vi "iFlex Open Lines.vi"(8 "error in (no error)":errorcluster) -> (0 "error out":errorcluster, 3 "iFlex Connected":bool, 5 "iFlex Control out":T1 {"Power 561" min=12.5 max=100.0 step=0.1 scale=0.0..100.0; "Power 488" min=30.0 max=100.0 step=0.1 scale=0.0..100.0})   [LabVIEW 2020]
uses:
  <vilib>/DAQmx/create/channels.llb/DAQmx Create Channel (DO-Digital Output).vi
  <vilib>/DAQmx/create/channels.llb/DAQmx Create Channel (AO-Voltage-Basic).vi
  _Controls/iFlex.ctl
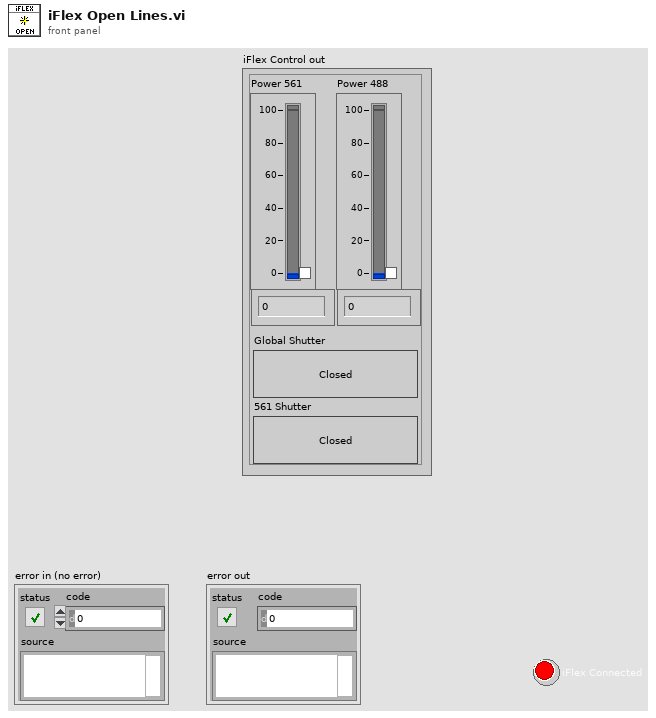
[diagram p1: front panel]
types:
  T1 = typedef "iFlex.ctl" = cluster{"Power 561":dbl, "Power 488":dbl, "Global Shutter":bool, "561 Shutter":bool}
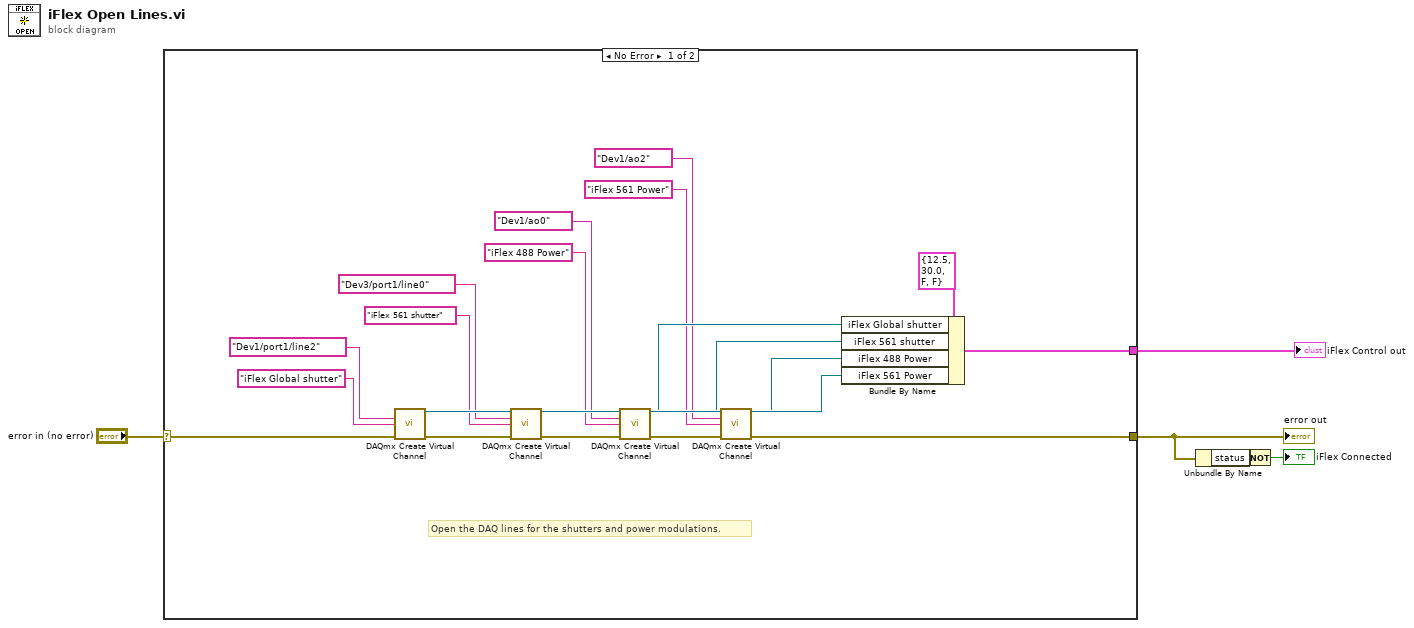
[diagram p0: block diagram]
diagram:
  n1 = case shown="No Error" "error in (no error)" {
    selector: "error in (no error)" -> [w7 w25]
    tunnel: [w24 w25] -> w3
    tunnel: [w23 _] -> w5
    frame No Error {
      # "Open the DAQ lines for the shutters and power modulations."
      n2 = call-poly <vilib>:"DAQmx Create Virtual Channel.vi"("lines"=tag "Dev1/port1/line2", "name to assign"="iFlex Global shutter", "error in"=w7) -> ("task out"=w19:refnum<k21>, "error out"=w16:errorcluster)  [unwired: 11 in]
      n3 = call-poly <vilib>:"DAQmx Create Virtual Channel.vi"("lines"=tag "Dev3/port1/line0", "name to assign"="iFlex 561 shutter", "error in"=w16) -> ("task out"=w20:refnum<k21>, "error out"=w17:errorcluster)  [unwired: 11 in]
      n4 = call-poly <vilib>:"DAQmx Create Virtual Channel.vi"("physical channels"=tag "Dev1/ao0", "name to assign"="iFlex 488 Power", "error in"=w17) -> ("task out"=w21:refnum<k21>, "error out"=w18:errorcluster)  [unwired: 11 in]
      n5 = call-poly <vilib>:"DAQmx Create Virtual Channel.vi"("physical channels"=tag "Dev1/ao2", "name to assign"="iFlex 561 Power", "error in"=w18) -> ("task out"=w22:refnum<k21>, "error out"=w24:errorcluster)  [unwired: 11 in]
      n6 = Bundle By Name(cluster=T1 {"Power 561"=12.5, "Power 488"=30.0, "Global Shutter"=FALSE, "561 Shutter"=FALSE} ("iFlex Control in"), "iFlex Global shutter"=w19, "iFlex 561 shutter"=w20, "iFlex 488 Power"=w21, "iFlex 561 Power"=w22) -> (w23:T1)
    }
    frame Error {
    }
  }
  "error out" <- w3
  "iFlex Control out" <- w5
  n7 = Unbundle By Name(w3) -> ("status"=w2:bool)
  n8 = Not(x=w2) -> (.not. x?=→"iFlex Connected":bool)
